vi "Ex-05 Acq Finite Multipoint FFT Noise&Sin Gen.vi"() -> ()   [LabVIEW 2012]
doc: "© Copyright M. Ferrari 2012\nMultipoint Analog Acq. Mean, FFT & Noise Gen"
uses:
  <vilib>/DAQmx/create/channels.llb/DAQmx Create Channel (AI-Voltage-Basic).vi
  <vilib>/DAQmx/configure/timing.llb/DAQmx Timing (Sample Clock).vi
  <vilib>/DAQmx/read.llb/DAQmx Read (Analog Wfm 1Chan NSamp).vi
  <vilib>/express/express analysis/Spectral/XNode/ExpressSpectralMeasurementsBlockNode.xnode
  <vilib>/express/express analysis/Spectral/Block/exnSpectralBlock spectral measurements RMS poly.vi
  <vilib>/express/express analysis/Spectral/Block/exnSpectralBlock spectral measurements RMS WFM.vi
  <vilib>/measure/NI_MABase.lvlib
panel:
  out "MEDIA":dbl format="%0.2f"
  in  "Amp. segnale Rif.":dbl(knob)=1.0 scale=0.0..5.0
  in  "Freq. segnale Rif.":dbl(knob)=100.0 scale=0.0..500.0
  in  "Ampiezza rumore":dbl(knob) scale=0.0..5.0
  in  "n° samples":i32=1000
  in  "rate":dbl=10000.0
  in  "min":dbl=-5.0 format="%0.2f"
  in  "max":dbl=5.0 format="%0.2f"
  in  "in conf":i32(ring)=10083 items=["default"=-1, "RSE"=10083, "NRSE"=10078, "Differential"=10106, "Pseudodifferential"=12529]
  in  "physical ch":tag="Dev1/ai0"
  out "FFT":cluster{"f0":dbl, "df":dbl, "magnitude":dbl[]}(graph)
  out "FFT - (RMS)":cluster{"f0":dbl, "df":dbl, "magnitude":dbl[]}
  out "Volt Graph":waveform(dbl)(graph)
  # "RANGE"
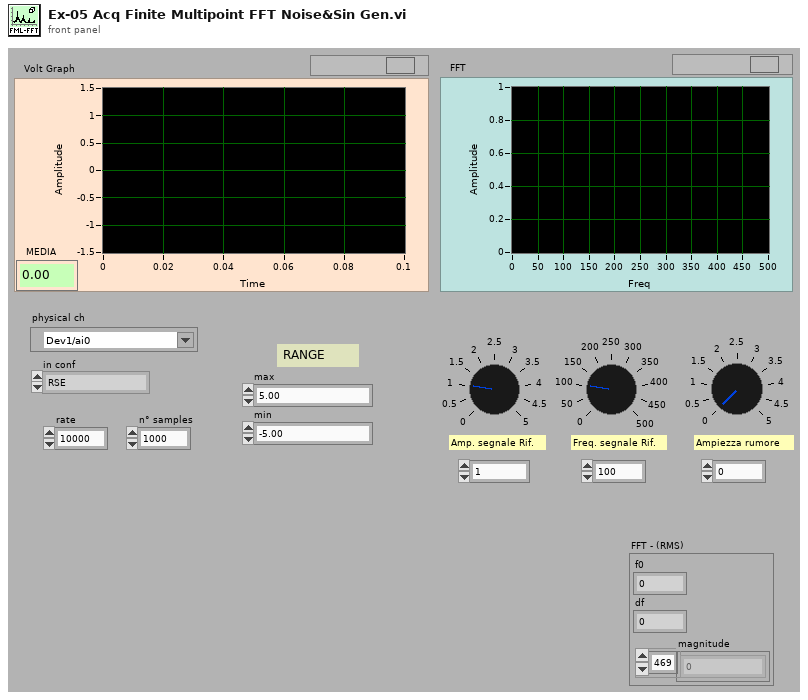
[diagram p1: front panel]
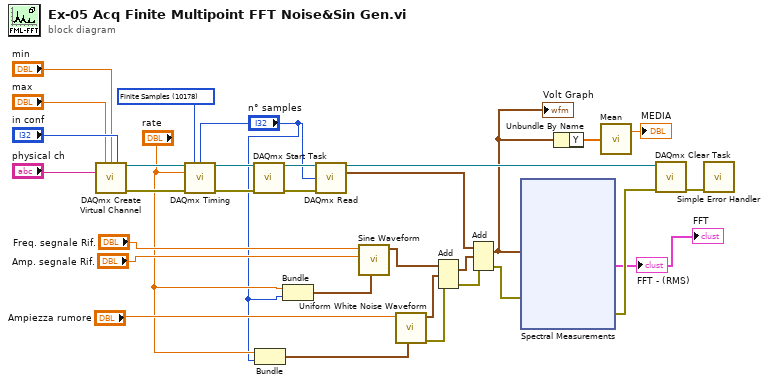
[diagram p0: block diagram]
diagram:
  w25 = 10178 items=["Finite Samples"=10178, "Continuous Samples"=10123, "Hardware Timed Single Point"=12522] ("sample mode")
  n1 = call-poly <vilib>:"DAQmx Create Virtual Channel.vi"("maximum value"="max", "minimum value"="min", "input terminal configuration"="in conf", "physical channels"="physical ch") -> ("task out"=w31:refnum<k21>, "error out"=w30:errorcluster)  [unwired: 5 in, 5 out]
  n2 = call-poly <vilib>:"DAQmx Timing.vi"("task/channels in"=w31, "sample mode"=w25, "samples per channel"="n° samples", "rate"="rate") -> ("task out"=w26:refnum<k21>)  [unwired: 3 in, 8 out]
  n3 = call <vilib>:"DAQmx Start Task.vi"("task/channels in"=w26, "error in"=w30) -> ("task out"=w29:refnum<k21>, "error out"=w28:errorcluster)  [unwired: 12 out]
  n4 = Bundle("rate"="rate", "n° samples"="n° samples") -> (w12:cluster{"rate":dbl, "n° samples":i32})  [unwired: 1 in]
  n5 = Bundle("rate"="rate", "n° samples"="n° samples") -> (w9:cluster{"rate":dbl, "n° samples":i32})  [unwired: 1 in]
  n6 = call-poly <vilib>:"DAQmx Read.vi"("task/channels in"=w29, "number of samples per channel"="n° samples", "error in"=w28) -> ("task out"=w27:refnum<k21>, "data"=w13:waveform(dbl))  [unwired: 11 out]
  n7 = call <vilib>:"Sine Waveform.vi"("sampling info"=w9, "amplitude"="Amp. segnale Rif.", "frequency"="Freq. segnale Rif.") -> ("signal out"=w6:waveform(dbl))  [unwired: 7 in, 1 out]
  n8 = call <vilib>:"Uniform White Noise Waveform.vi"("sampling info"=w12, "amplitude"="Ampiezza rumore") -> ("error out"=w3:errorcluster, "signal out"=w7:waveform(dbl))  [unwired: 3 in, 5 out]
  n9 = Add(1:w7, 2:w6, 4:w3) -> (0:w8:waveform(dbl), 3:w5:errorcluster)
  n10 = Add(1:w8, 2:w13, 4:w5) -> (0:w14:waveform(dbl), 3:w4:errorcluster)
  "Volt Graph" <- w14
  n11 = xnode "Spectral Measurements"("Signals"=w14, "error in (no error)"=w4) -> ("FFT - (RMS)"=→"FFT - (RMS)" →"FFT":cluster{"f0":dbl, "df":dbl, "magnitude":dbl[]}, "error out"=w21:errorcluster)  [unwired: 1 out]
  n12 = Unbundle By Name(w14) -> ("Y"=w22:dbl[])
  n13 = call <vilib>:"Mean.vi"("X"=w22) -> ("mean"=→"MEDIA":dbl)  [unwired: 1 out]
  n14 = call <vilib>:"DAQmx Clear Task.vi"("task in"=w27, "error in"=w21) -> ("error out"=w24:errorcluster)  [unwired: 13 out]
  n15 = call <vilib>:"Simple Error Handler.vi"("error in (no error)"=w24) -> ()  [unwired: 1 in, 8 out]
